vi "sphere tracking settings from scan settings.vi"(6 "gaussian":bool, 7 "sphere radius/sigma":u16, 9 "Vdiff /(g^2*1ms)":dbl=0.01, 10 "scan specification":T1) -> (2 "tracking settings out":T2={"scan radius"=0, "2^16/lines per revolution"=1394, "gx"=0.0, "rtw"=0.0, "lines per revolution"=47, "vel diff"=0.0})   [LabVIEW 2010]
uses:
  FPGA tracking/polar tracking settings.ctl
  scan_specification_tagResonant.ctl
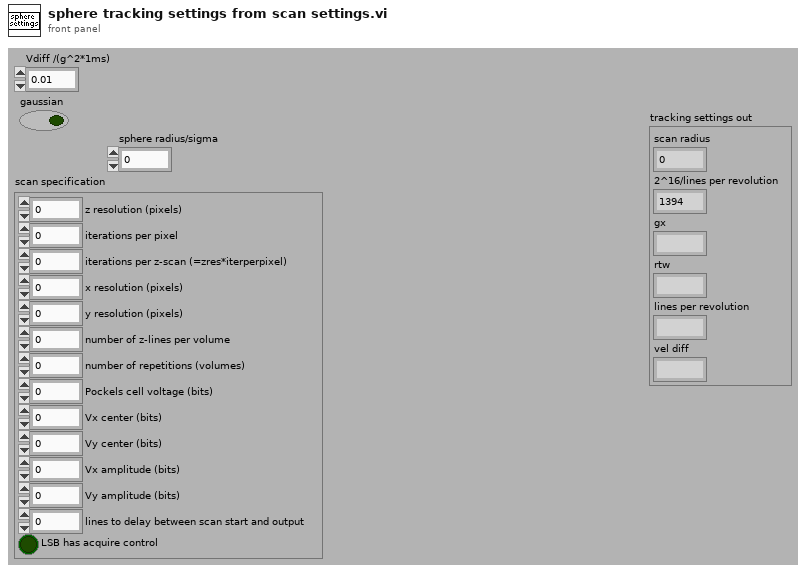
[diagram p1: front panel]
types:
  T1 = typedef "scan_specification_tagResonant.ctl" = cluster{"z resolution (pixels)":u16, "iterations per pixel":u16, "iterations per z-scan (=zres*iterperpixel)":u16, "x resolution (pixels)":u16, "y resolution (pixels)":u16, "number of z-lines per volume":u16, "number of repetitions (volumes)":i32, "Pockels cell voltage (bits)":i16, "Vx center (bits)":i16, "Vy center (bits)":i16, "Vx amplitude (bits)":i16, "Vy amplitude (bits)":i16, "lines to delay between scan start and output":u16, "LSB has acquire control":bool}
  T2 = typedef "polar tracking settings.ctl" = cluster{"scan radius":u16, "2^16/lines per revolution":u16, "gx":fxp<+,16,8>, "rtw":fxp<+,16,26>, "lines per revolution":u8, "vel diff":fxp<+,24,-22>}
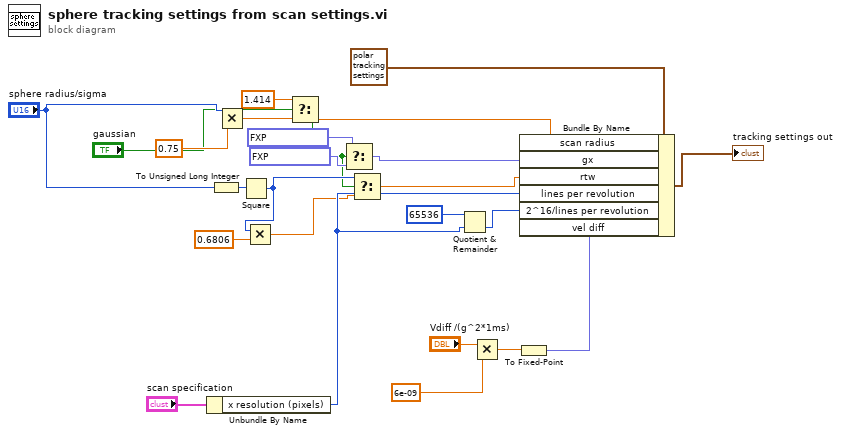
[diagram p0: block diagram]
diagram:
  n1 = Unbundle By Name("scan specification") -> ("x resolution (pixels)"=w15:u16)
  n2 = To Unsigned Long Integer(number="sphere radius/sigma") -> (unsigned 32bit integer=w19:u32)
  n3 = Multiply(x="sphere radius/sigma", y=0.75) -> (x*y=w22:dbl)
  n4 = Square(x=w19) -> (x^2=w3:u32)
  n5 = Multiply(x=w3, y=0.6806) -> (x*y=w4:dbl)
  n6 = Select(t=1.414, s="gaussian", f=w22) -> (s? t:f=w9:dbl)
  n7 = Select(t=fxp<+,16,8> 1.0, s="gaussian", f=fxp<+,16,8> 1.5546875 ("gx")) -> (s? t:f=w6:fxp<+,16,8>)
  n8 = Select(t=w3, s="gaussian", f=w4) -> (s? t:f=w1:dbl)
  n9 = Quotient & Remainder(x=65536, y=w15) -> (floor(x/y)=w14:i32)  [unwired: 1 out]
  n10 = Multiply(x="Vdiff /(g^2*1ms)", y=6e-09) -> (x*y=w11:dbl)
  n11 = To Fixed-Point(number=w11) -> (fixed-point=w10:fxp<+,24,-22>)  [unwired: 1 in]
  n12 = Bundle By Name(cluster=T2 {"scan radius"=0, "2^16/lines per revolution"=1394, "gx"=0.0, "rtw"=0.0, "lines per revolution"=47, "vel diff"=0.0} ("tracking settings"), "scan radius"=w9, "gx"=w6, "rtw"=w1, "lines per revolution"=w15, "2^16/lines per revolution"=w14, "vel diff"=w10) -> (→"tracking settings out":T2)
